vi "Galil_commandValue.vi"() -> ()   [LabVIEW 2010]
panel:
  in  "Galil.IGalil":refnum<k7>
  out "Library Version:":string
  out "Response":dbl
  in  "Command:":string
  out "error out":errorcluster
  out "Connected To:":string
  in  "Connection String:":string
  # "This vi Shows how to use the commandValue function in the Galil Communications Library.  \n\nIf Connection String is left blank, the vi will open the connections dialog when run.  If a value is input into Connection String, the vi will attempt to connect to the controller at that address (ex COM1 19200).\n\nInsert a Galil Command into the Command: box (ex MG TIME), when the vi is run, that command will be sent to the controller and the response is shown in the Response: box."
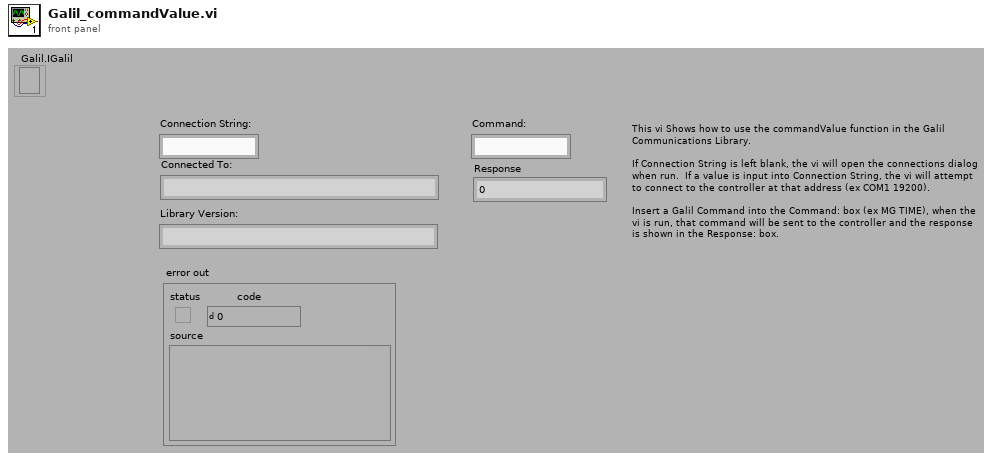
[diagram p1: front panel]
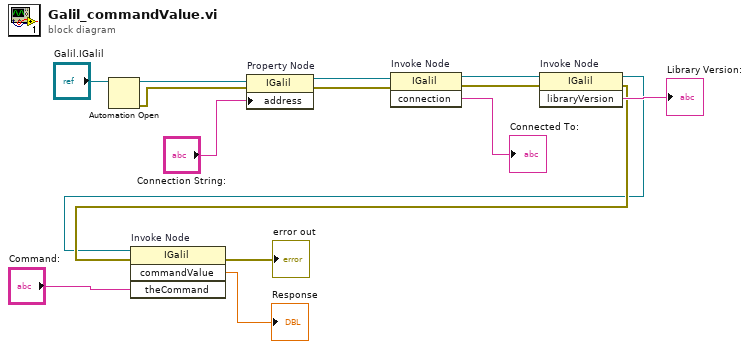
[diagram p0: block diagram]
diagram:
  n1 = Automation Open(Automation Refnum="Galil.IGalil") -> (Automation Refnum=w15:refnum<k7>, error out=w13:errorcluster)  [unwired: 1 in, 2 out]
  n2 = property on="Property Node" class="IGalil"(reference=w15, error in=w13, "address"="Connection String:") -> (reference out=w14:refnum<k7>, error out=w12:errorcluster)
  n3 = invoke on="Invoke Node" class="IGalil" method="connection"(reference=w14, error in=w12) -> (reference out=w7:refnum<k7>, error out=w6:errorcluster, "connection"=→"Connected To:":string)  [unwired: 1 in]
  n4 = invoke on="Invoke Node" class="IGalil" method="libraryVersion"(reference=w7, error in=w6) -> (reference out=w3:refnum<k7>, error out=w4:errorcluster, "libraryVersion"=→"Library Version:":string)  [unwired: 1 in]
  n5 = invoke on="Invoke Node" class="IGalil" method="commandValue"(reference=w3, error in=w4, "theCommand"="Command:") -> (error out=→"error out":errorcluster, "commandValue"=→"Response":dbl)  [unwired: 1 in, 2 out]
